vi "Set IP Address.vi"(8 "error in (no error)":errorcluster, 10 "IP Address":string, 11 "ENET in":refnum<class "ENET_BS1201.lvclass">) -> (0 "error out":errorcluster, 3 "ENET out":refnum<class "ENET_BS1201.lvclass">)   [LabVIEW 2021, in "BS120x Driver.lvlib" / "ENET_BS1201.lvclass"]
uses:
  ENET_BS1201.lvclass
  C:/Users/Public/Documents/Projects/7100-00109 SW BS1201 LV Driver/trunk/source/ENET_BS120x/ENET_BS120x.lvclass
  <vilib>/regexp/Match Regular Expression.xnode
  ENET_BS120x/ENET_BS120x.lvclass
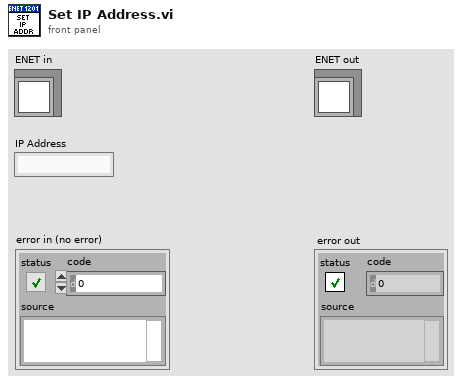
[diagram p1: front panel]
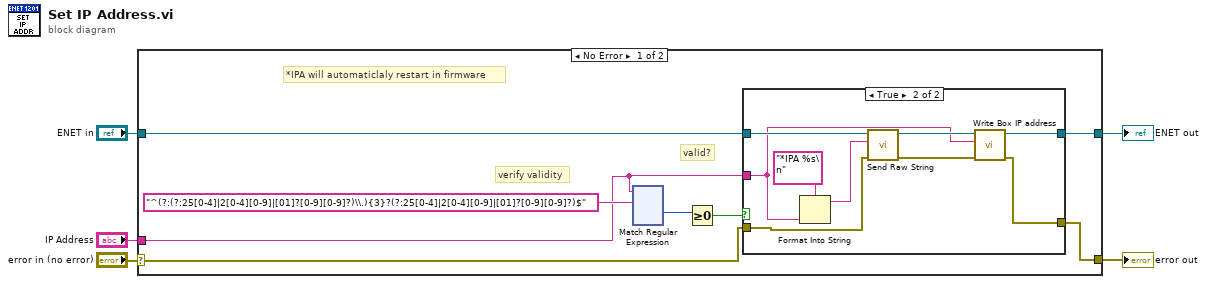
[diagram p0: block diagram]
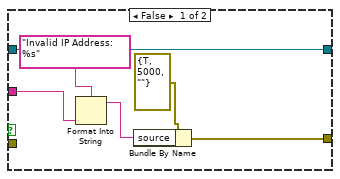
[diagram p2: hidden frame]
diagram:
  n1 = case shown="No Error" "error in (no error)" {
    selector: "error in (no error)" -> [w7 w147]
    tunnel: [w6 w147] -> w5
    tunnel: [w8 w146] -> w4
    tunnel: "ENET in" -> [w13 w146]
    tunnel: "IP Address" -> [w9 _]
    frame No Error {
      # "*IPA will automaticlaly restart in firmware"
      # "valid?"
      # "verify validity"
      n2 = xnode "Match Regular Expression"("input string"=w9, "regular expression"="^(?:(?:25[0-4]|2[0-4][0-9]|[01]?[0-9][0-9]?)\\.){3}?(?:25[0-4]|2[0-4][0-9]|[01]?[0-9][0-9]?)$") -> ("offset past match"=w11:i32)  [unwired: 4 in, 4 out]
      n3 = Greater Or Equal To 0?(x=w11) -> (x >= 0?=w10:bool)
      n4 = case shown="True" w10 {
        tunnel: w13 -> [w19 w28]
        tunnel: w9 -> [w17 w22]
        tunnel: [w19 w23] -> w8
        tunnel: w7 -> [_ w25]
        tunnel: [w14 w20] -> w6
        frame False {
          n5 = Format Into String(format string="Invalid IP Address: %s", w17) -> (resulting string=w15:string)  [unwired: 2 in, 1 out]
          n6 = Bundle By Name(cluster=errorcluster {"status"=TRUE, "code"=5000, "source"=""} ("error out"), "source"=w15) -> (w14:errorcluster)
        }
        frame True {
          n7 = Format Into String(format string="*IPA %s\n", w22) -> (resulting string=w26:string)  [unwired: 2 in, 1 out]
          n8 = call "Send Raw String.vi"("error in (no error)"=w25, "String Data"=w26, "ENET in"=w28) -> ("error out"=w21:errorcluster, "ENET out"=w24:refnum<class "ENET_BS1201.lvclass">)  [unwired: 7 in]
          n9 = call-dynamic "Write Box IP address.vi"("error in (no error)"=w21, "Box IP address"=w22, "ENET_BS120x in"=w24) -> ("error out"=w20:errorcluster, "ENET_BS120x out"=w23:refnum<class "ENET_BS1201.lvclass">)  [unwired: 7 in]
        }
      }
    }
    frame Error {
    }
  }
  "error out" <- w5
  "ENET out" <- w4
